vi "Circ Line Filter 2.vi"(5 "Filter On?":bool, 8 "error in":errorcluster, 11 "Data Cluster In":T1={"Display X"=[], "Display Y"=[], "Encoder"=[], "Phi Array"=[], "Active Channel"=0, "Raw X"=[], "Raw Y"=[], "IIR filter specifications"={"Topology"=enum."Butterworth", "Type"=enum."Lowpass", "Order"=1, "Lower Fc"=20.0, "Upper Fc"=200.0, "PB Ripple"=1.0, "SB Attenuation"=60.0}, "Sample Rate"=100.0, "optional IIR filter specifications"={"Lower PB"=100.0, "Upper PB"=0.0, "Lower SB"=200.0, "Upper SB"=0.0, "PB Gain"=-3.0, "SB Gain"=-60.0, "Scale"=TRUE}, "Display Select"=enum."Locations", "Cursor Position"=0.0, "Position Mark"=[], "Window Size"=0.0, "Last Active Channel"=0, "Rotate to:"=0.0, "Averaged Locations"=[], "Scale Factors"=[], "Filtered Data Measurements"={"Vpp"=0.0, "Phase"=0.0, "Slope"=0.0, "Start Point"={[], []}, "End Point"={[], []}, "Slope Points"={"x1"=0.0, "y1"=0.0, "x2"=0.0, "y2"=0.0}}, "Mp Flag"=FALSE, "Number of Channels"=0, "NormVals"=[], "Norm Buffer"=[], "Current Assignments"=[], "Current Filter Response"={"t0"=timestamp(0 s since 1904-01-01), "dt"=0.0, "Y"=[]}, "Filter Coeffs"=[], "Strip Data"=[], "X Display Null"=[], "Y Display Null"=[], "X Display Null Mod"=[], "Y Display Null Mod"=[], "file names"=[], "Current Data File"="", "Current Data Path"=path "", "Slide Value"=0, "Setup File Path"=path "", "Plot Color"=[], "Start Pts"=[], "End Pts"=[], "Slope Points"=[], "Raw Data Measurements"={"Vpp"=0.0, "Phase"=0.0, "Slope"=0.0, "Start Point"={[], []}, "End Point"={[], []}, "Slope Points"={"x1"=0.0, "y1"=0.0, "x2"=0.0, "y2"=0.0}}, "Raw Data"=refnum, "Calc X"=[], "Calc Y"=[], "3D X"=refnum, "3D Y"=refnum, "C/L Filter X  Waveforms"=[], "C/L Filter Y Waveforms"=[], "Command History"=[], "Filter Flag"={"Last Setter"="", "Status"=FALSE}, "Phi Array Scratch"=[], "Filetype"=enum."20\" Tool", "Channel List"={"Channel 1"=FALSE, "Channel 2"=FALSE, "Channel 3"=FALSE, "Channel 4"=FALSE, "Channel 5"=FALSE, "Channel 6"=FALSE, "Channel 7"=FALSE, "Channel 8"=FALSE, "Channel 9"=FALSE, "Channel 10"=FALSE, "Channel 11"=FALSE, "Channel 12"=FALSE, "Channel 13"=FALSE, "Channel 14"=FALSE, "Channel 15"=FALSE, "Channel 16"=FALSE, "Channel 17"=FALSE, "Channel 18"=FALSE, "Channel 19"=FALSE, "Channel 20"=FALSE, "Channel 21"=FALSE, "Channel 22"=FALSE, "Channel 23"=FALSE, "Channel 24"=FALSE, "Channel 25"=FALSE, "Channel 26"=FALSE, "Channel 27"=FALSE, "Channel 28"=FALSE, "Channel 29"=FALSE, "Channel 30"=FALSE, "Channel 31"=FALSE, "Channel 32"=FALSE}, "Channel Indicies"=[], "Calc Raw X"=[], "Calc Raw Y"=[], "Old Channel Indicies"=[]} {"Rotate to:" items=["1", "2", "3", "4", "5", "6", "7", "8", "9", "10", "11", "12", "3", "4", "15", "16", "17", "18", "19", "20", "21", "22", "23", "24"]; "Last Active Channel" items=["1", "2", "3", "4", "5", "6", "7", "8", "9", "10", "11", "12", "3", "4", "15", "16", "17", "18", "19", "20", "21", "22", "23", "24"]; "optional IIR filter specifications"."PB Gain" format="%0.2f"; "optional IIR filter specifications"."SB Gain" format="%0.2f"; "optional IIR filter specifications"."Lower SB" format="%0.2p"; "optional IIR filter specifications"."Upper SB" format="%0.2f"; "optional IIR filter specifications"."Lower PB" format="%0.2p"; "optional IIR filter specifications"."Upper PB" format="%0.2f"; "IIR filter specifications"."PB Ripple" format="%0.2f"; "IIR filter specifications"."Lower Fc" format="%0.2p"; "IIR filter specifications"."SB Attenuation" format="%0.2f"; "IIR filter specifications"."Upper Fc" format="%0.2p"; "Active Channel" items=["1", "2", "3", "4", "5", "6", "7", "8", "9", "10", "11", "12", "3", "4", "15", "16", "17", "18", "19", "20", "21", "22", "23", "24"]}) -> (0 "error out":errorcluster, 3 "Data Cluster Out":T1={"Display X"=[], "Display Y"=[], "Encoder"=[], "Phi Array"=[], "Active Channel"=0, "Raw X"=[], "Raw Y"=[], "IIR filter specifications"={"Topology"=enum."Butterworth", "Type"=enum."Lowpass", "Order"=1, "Lower Fc"=20.0, "Upper Fc"=200.0, "PB Ripple"=1.0, "SB Attenuation"=60.0}, "Sample Rate"=100.0, "optional IIR filter specifications"={"Lower PB"=100.0, "Upper PB"=0.0, "Lower SB"=200.0, "Upper SB"=0.0, "PB Gain"=-3.0, "SB Gain"=-60.0, "Scale"=TRUE}, "Display Select"=enum."Locations", "Cursor Position"=0.0, "Position Mark"=[], "Window Size"=0.0, "Last Active Channel"=0, "Rotate to:"=0.0, "Averaged Locations"=[], "Scale Factors"=[], "Filtered Data Measurements"={"Vpp"=0.0, "Phase"=0.0, "Slope"=0.0, "Start Point"={[], []}, "End Point"={[], []}, "Slope Points"={"x1"=0.0, "y1"=0.0, "x2"=0.0, "y2"=0.0}}, "Mp Flag"=FALSE, "Number of Channels"=0, "NormVals"=[], "Norm Buffer"=[], "Current Assignments"=[], "Current Filter Response"={"t0"=timestamp(0 s since 1904-01-01), "dt"=0.0, "Y"=[]}, "Filter Coeffs"=[], "Strip Data"=[], "X Display Null"=[], "Y Display Null"=[], "X Display Null Mod"=[], "Y Display Null Mod"=[], "file names"=[], "Current Data File"="", "Current Data Path"=path "", "Slide Value"=0, "Setup File Path"=path "", "Plot Color"=[], "Start Pts"=[], "End Pts"=[], "Slope Points"=[], "Raw Data Measurements"={"Vpp"=0.0, "Phase"=0.0, "Slope"=0.0, "Start Point"={[], []}, "End Point"={[], []}, "Slope Points"={"x1"=0.0, "y1"=0.0, "x2"=0.0, "y2"=0.0}}, "Raw Data"=refnum, "Calc X"=[], "Calc Y"=[], "3D X"=refnum, "3D Y"=refnum, "C/L Filter X  Waveforms"=[], "C/L Filter Y Waveforms"=[], "Command History"=[], "Filter Flag"={"Last Setter"="", "Status"=FALSE}, "Phi Array Scratch"=[], "Filetype"=enum."20\" Tool", "Channel List"={"Channel 1"=FALSE, "Channel 2"=FALSE, "Channel 3"=FALSE, "Channel 4"=FALSE, "Channel 5"=FALSE, "Channel 6"=FALSE, "Channel 7"=FALSE, "Channel 8"=FALSE, "Channel 9"=FALSE, "Channel 10"=FALSE, "Channel 11"=FALSE, "Channel 12"=FALSE, "Channel 13"=FALSE, "Channel 14"=FALSE, "Channel 15"=FALSE, "Channel 16"=FALSE, "Channel 17"=FALSE, "Channel 18"=FALSE, "Channel 19"=FALSE, "Channel 20"=FALSE, "Channel 21"=FALSE, "Channel 22"=FALSE, "Channel 23"=FALSE, "Channel 24"=FALSE, "Channel 25"=FALSE, "Channel 26"=FALSE, "Channel 27"=FALSE, "Channel 28"=FALSE, "Channel 29"=FALSE, "Channel 30"=FALSE, "Channel 31"=FALSE, "Channel 32"=FALSE}, "Channel Indicies"=[], "Calc Raw X"=[], "Calc Raw Y"=[], "Old Channel Indicies"=[]} {"Rotate to:" items=["1", "2", "3", "4", "5", "6", "7", "8", "9", "10", "11", "12", "3", "4", "15", "16", "17", "18", "19", "20", "21", "22", "23", "24"]; "Last Active Channel" items=["1", "2", "3", "4", "5", "6", "7", "8", "9", "10", "11", "12", "3", "4", "15", "16", "17", "18", "19", "20", "21", "22", "23", "24"]; "optional IIR filter specifications"."PB Gain" format="%0.2f"; "optional IIR filter specifications"."SB Gain" format="%0.2f"; "optional IIR filter specifications"."Lower SB" format="%0.2p"; "optional IIR filter specifications"."Upper SB" format="%0.2f"; "optional IIR filter specifications"."Lower PB" format="%0.2p"; "optional IIR filter specifications"."Upper PB" format="%0.2f"; "IIR filter specifications"."PB Ripple" format="%0.2f"; "IIR filter specifications"."Lower Fc" format="%0.2p"; "IIR filter specifications"."SB Attenuation" format="%0.2f"; "IIR filter specifications"."Upper Fc" format="%0.2p"; "Active Channel" items=["1", "2", "3", "4", "5", "6", "7", "8", "9", "10", "11", "12", "3", "4", "15", "16", "17", "18", "19", "20", "21", "22", "23", "24"]})   [LabVIEW 2017]
uses:
  <vilib>/Analysis/NI_AALPro.lvlib
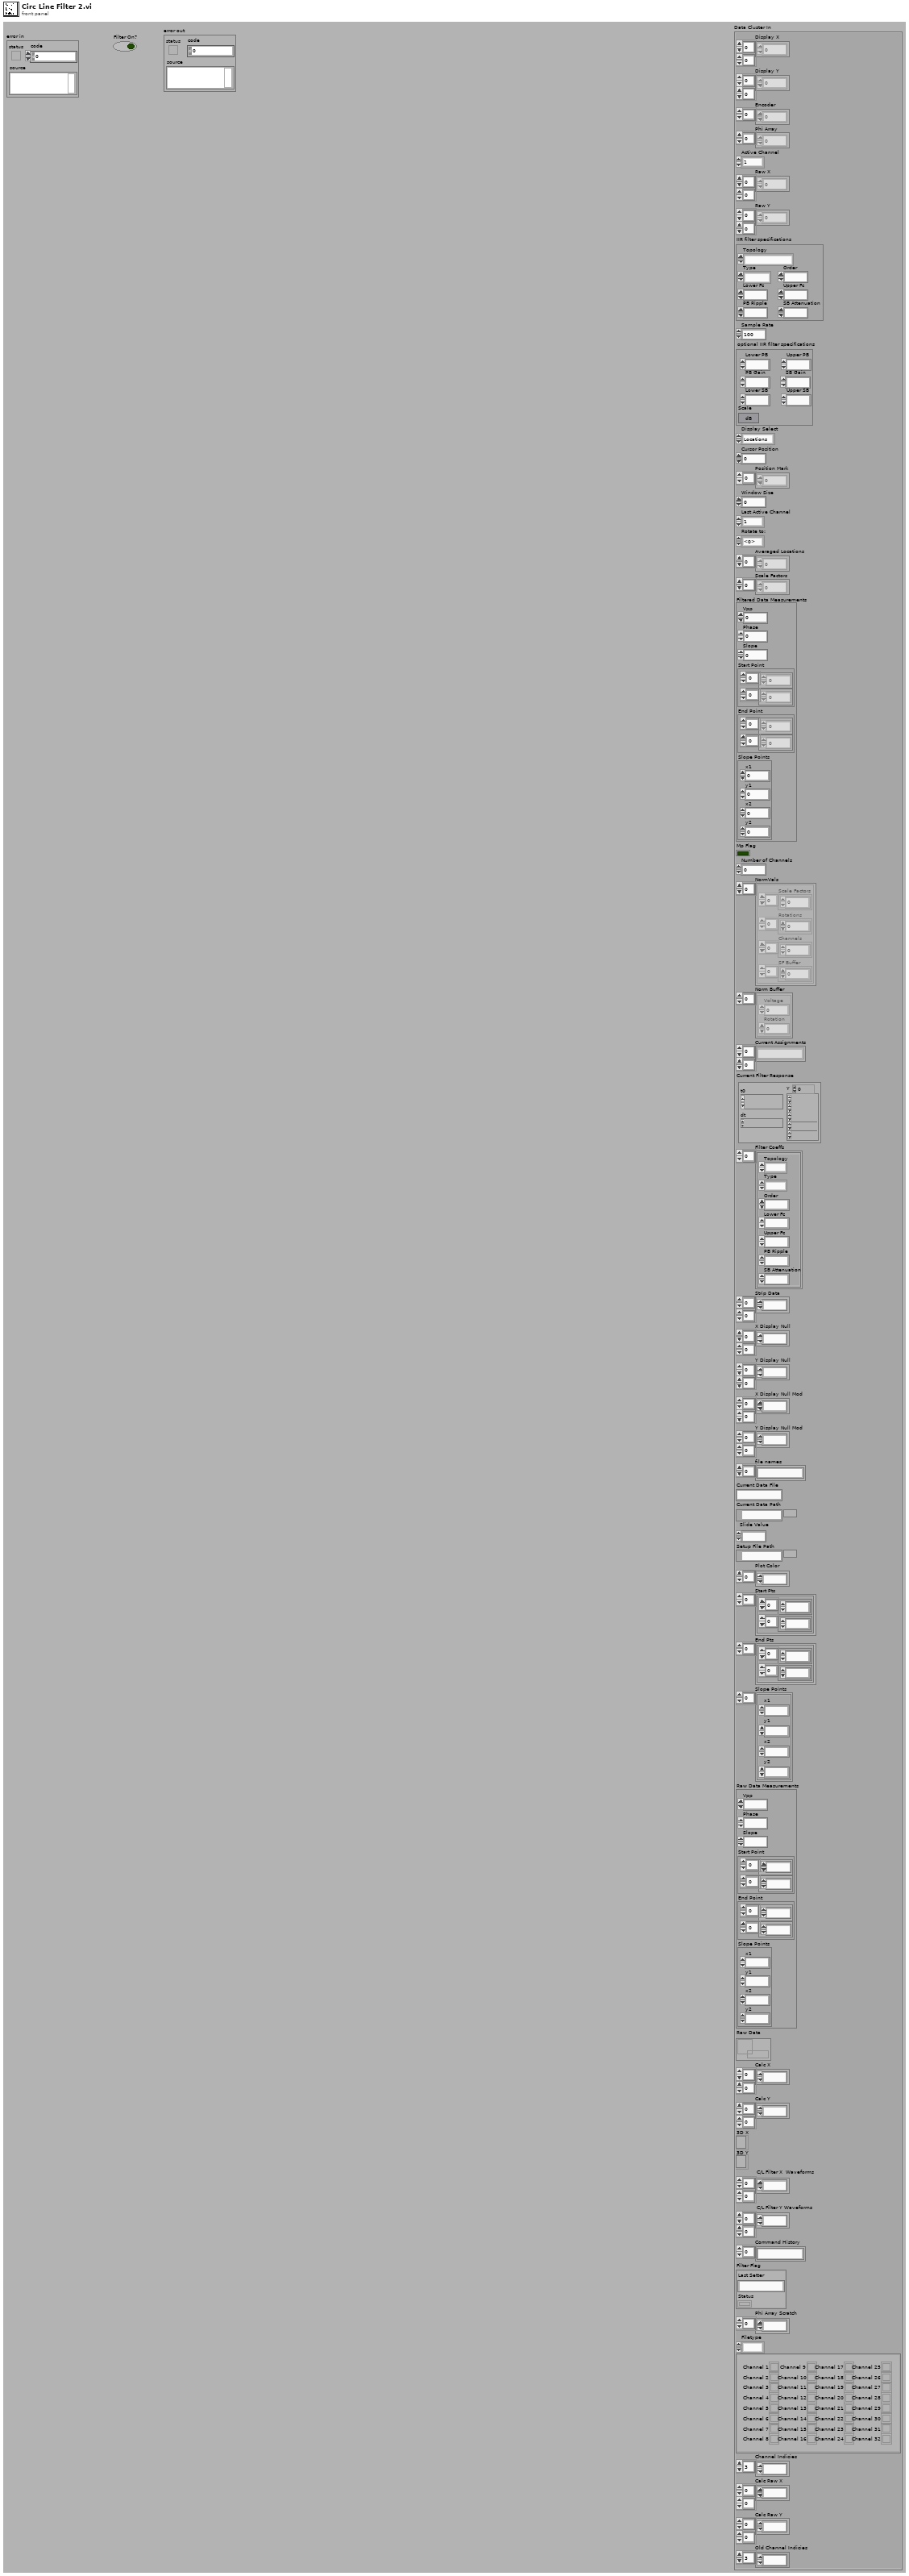
[diagram p1: front panel]
types:
  T1 = cluster{"Display X":dbl[][], "Display Y":dbl[][], "Encoder":dbl[], "Phi Array":dbl[], "Active Channel":i32, "Raw X":dbl[][], "Raw Y":dbl[][], "IIR filter specifications":cluster{"Topology":enum16{"Off", "Butterworth", "Chebyshev", "Inverse Chebyshev", "Elliptic", "Bessel"}, "Type":enum16{"Lowpass", "Highpass", "Bandpass", "Bandstop"}, "Order":i32, "Lower Fc":dbl, "Upper Fc":dbl, "PB Ripple":dbl, "SB Attenuation":dbl}, "Sample Rate":dbl, "optional IIR filter specifications":cluster{"Lower PB":dbl, "Upper PB":dbl, "Lower SB":dbl, "Upper SB":dbl, "PB Gain":dbl, "SB Gain":dbl, "Scale":bool}, "Display Select":enum32{"Channel Detail", "X Strip", "Y Strip", "Locations", "Contour", "3D", "Sorted"}, "Cursor Position":dbl, "Position Mark":sgl[], "Window Size":dbl, "Last Active Channel":i32, "Rotate to:":dbl, "Averaged Locations":i32[], "Scale Factors":dbl[], "Filtered Data Measurements":cluster{"Vpp":dbl, "Phase":dbl, "Slope":dbl, "Start Point":cluster{dbl[], dbl[]}, "End Point":cluster{dbl[], dbl[]}, "Slope Points":cluster{"x1":dbl, "y1":dbl, "x2":dbl, "y2":dbl}}, "Mp Flag":bool, "Number of Channels":i32, "NormVals":cluster{"Scale Factors":dbl[], "Rotations":dbl[], "Channels":i32[], "SF Buffer":dbl[]}[], "Norm Buffer":cluster{"Voltage":dbl, "Rotation":dbl}[], "Current Assignments":string[][], "Current Filter Response":waveform(dbl), "Filter Coeffs":cluster{"Topology":enum16{"Off", "Butterworth", "Chebyshev", "Inverse Chebyshev", "Elliptic", "Bessel"}, "Type":enum16{"Lowpass", "Highpass", "Bandpass", "Bandstop"}, "Order":i32, "Lower Fc":dbl, "Upper Fc":dbl, "PB Ripple":dbl, "SB Attenuation":dbl}[], "Strip Data":dbl[][], "X Display Null":dbl[][], "Y Display Null":dbl[][], "X Display Null Mod":dbl[][], "Y Display Null Mod":dbl[][], "file names":string[], "Current Data File":string, "Current Data Path":path, "Slide Value":i32, "Setup File Path":path, "Plot Color":i32[], "Start Pts":cluster{dbl[], dbl[]}[], "End Pts":cluster{dbl[], dbl[]}[], "Slope Points":cluster{"x1":dbl, "y1":dbl, "x2":dbl, "y2":dbl}[], "Raw Data Measurements":cluster{"Vpp":dbl, "Phase":dbl, "Slope":dbl, "Start Point":cluster{dbl[], dbl[]}, "End Point":cluster{dbl[], dbl[]}, "Slope Points":cluster{"x1":dbl, "y1":dbl, "x2":dbl, "y2":dbl}}, "Raw Data":refnum<queue>, "Calc X":dbl[][], "Calc Y":dbl[][], "3D X":refnum<k7>, "3D Y":refnum<k7>, "C/L Filter X  Waveforms":dbl[][], "C/L Filter Y Waveforms":dbl[][], "Command History":string[], "Filter Flag":cluster{"Last Setter":string, "Status":bool}, "Phi Array Scratch":dbl[], "Filetype":enum16{"20\" Tool", "24\"/36\" Tool"}, "Channel List":cluster{"Channel 1":bool, "Channel 2":bool, "Channel 3":bool, "Channel 4":bool, "Channel 5":bool, "Channel 6":bool, "Channel 7":bool, "Channel 8":bool, "Channel 9":bool, "Channel 10":bool, "Channel 11":bool, "Channel 12":bool, "Channel 13":bool, "Channel 14":bool, "Channel 15":bool, "Channel 16":bool, "Channel 17":bool, "Channel 18":bool, "Channel 19":bool, "Channel 20":bool, "Channel 21":bool, "Channel 22":bool, "Channel 23":bool, "Channel 24":bool, "Channel 25":bool, "Channel 26":bool, "Channel 27":bool, "Channel 28":bool, "Channel 29":bool, "Channel 30":bool, "Channel 31":bool, "Channel 32":bool}, "Channel Indicies":i32[], "Calc Raw X":dbl[][], "Calc Raw Y":dbl[][], "Old Channel Indicies":i32[]}
  T2 = enum32{"SVD", "Givens", "Givens2", "Householder", "LU Decomposition", "Cholesky"}
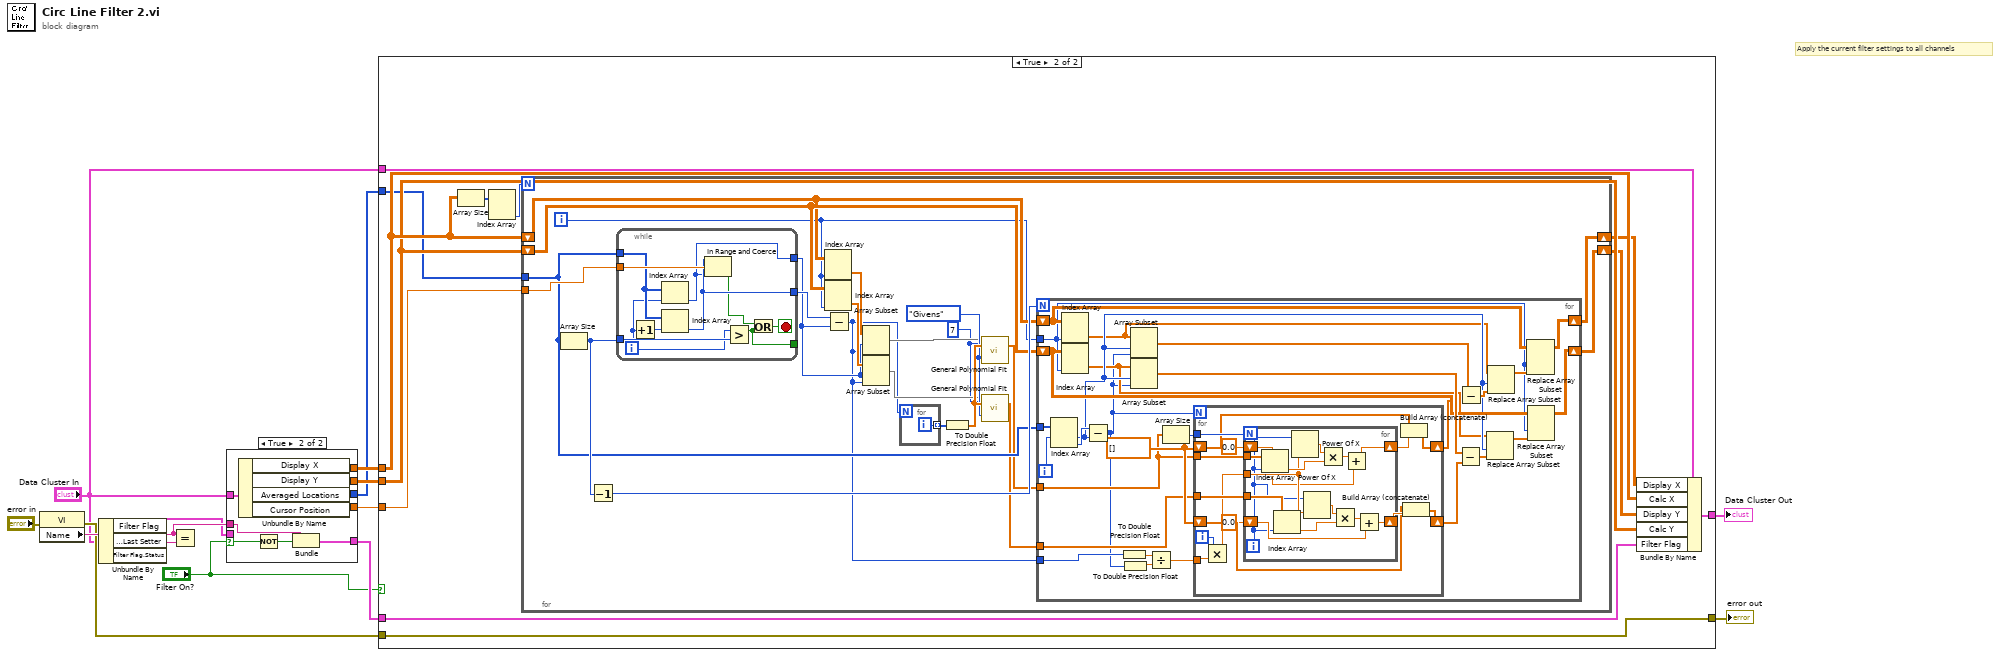
[diagram p0: block diagram]
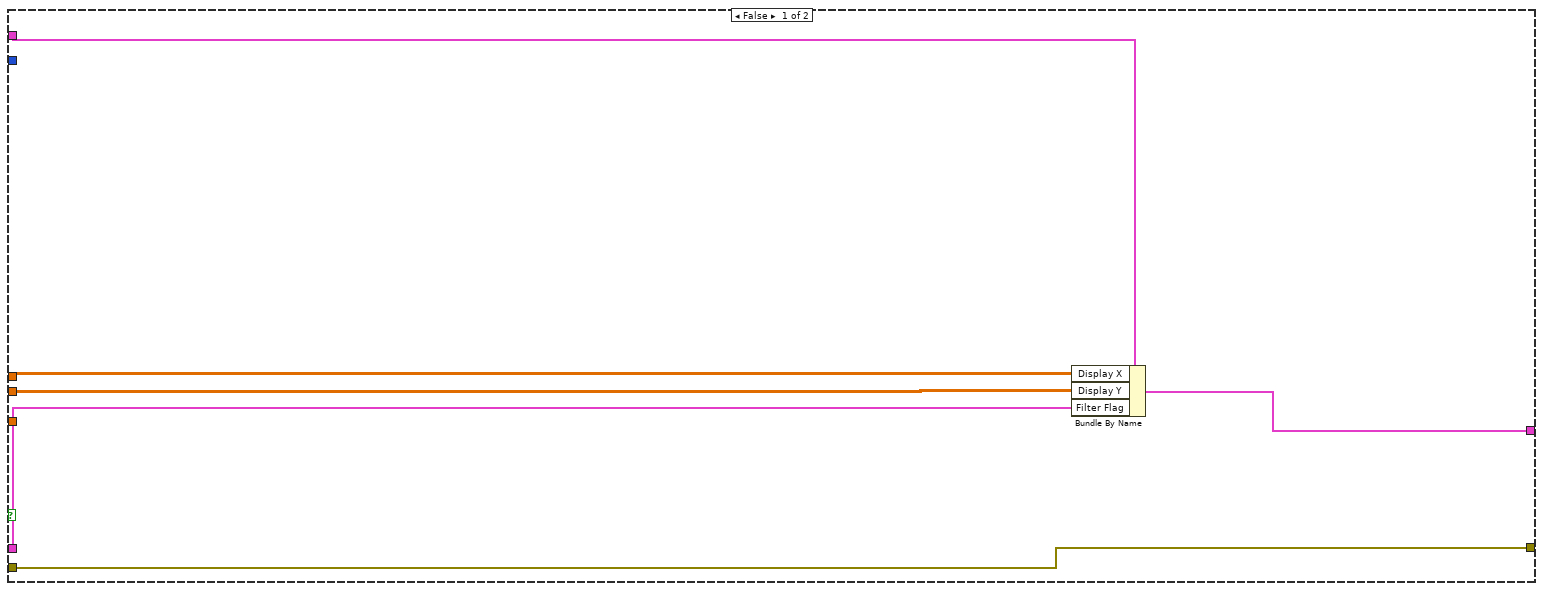
[diagram p2: hidden frame]
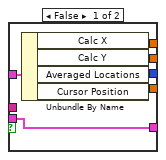
[diagram p3: hidden frame]
diagram:
  # "Apply the current filter settings to all channels"
  n1 = property class="VI"(error in="error in") -> (error out=w5:errorcluster, "Name"=w6:string)  [unwired: 1 in, 1 out]
  n2 = Unbundle By Name("Data Cluster In") -> ("Filter Flag"=w4:cluster{"Last Setter":string, "Status":bool}, "Filter Flag.Last Setter"=w8:string)  [unwired: 1 out]
  n3 = Equal?(x=w6, y=w8) -> ()  [unwired: 1 out]
  n4 = case shown="True" "Filter On?" {
    selector: "Filter On?" -> [_ w25]
    tunnel: "Data Cluster In" -> [w20 w29]
    tunnel: [w19 w28] -> w14
    tunnel: [w18 w27] -> w13
    tunnel: [w17 w26] -> w12
    tunnel: [w16 w21] -> w10
    tunnel: [w15 w22] -> w9
    tunnel: w6 -> [_ w24]
    tunnel: w4 -> [w15 _]
    frame False {
      n5 = Unbundle By Name(w20) -> ("Calc X"=w17:dbl[][], "Calc Y"=w18:dbl[][], "Averaged Locations"=w16:i32[], "Cursor Position"=w19:dbl)
    }
    frame True {
      n6 = Unbundle By Name(w29) -> ("Display X"=w26:dbl[][], "Display Y"=w27:dbl[][], "Averaged Locations"=w21:i32[], "Cursor Position"=w28:dbl)
      n7 = Not(x=w25) -> (.not. x?=w23:bool)
      n8 = Bundle("Name"=w24, w23) -> (w22:cluster{"Name":string, bool})  [unwired: 1 in]
    }
  }
  n9 = case shown="True" "Filter On?" {
    tunnel: w14 -> [_ w39]
    tunnel: w13 -> [w33 w41]
    tunnel: w12 -> [w34 w42]
    tunnel: [w35 w36] -> w11
    tunnel: w5 -> [w35 w36]
    tunnel: w10 -> [_ w40]
    tunnel: w9 -> [w31 w45]
    tunnel: "Data Cluster In" -> [w32 w47]
    tunnel: [w30 w46] -> w2
    frame False {
      n10 = Bundle By Name(cluster=w32, "Display X"=w34, "Display Y"=w33, "Filter Flag"=w31) -> (w30:T1)
    }
    frame True {
      n11 = Array Size(array=w42) -> (size(s)=w44:i32[])
      n12 = Index Array(array=w44) -> (element #2=w43:i32)  [unwired: 2 in, 1 out]
      n13 = for {
        N: w43 -> [_]
        tunnel: w39 -> [w69]
        tunnel: w40 -> [w57]
        shift-right: [w49] -> w38
        shift-left: w42 -> [w51]
        shift-right: [w48] -> w37
        shift-left: w41 -> [w56]
        i -> [w50]
        w66 = T2."Givens" ("algorithm")
        w60 = 7 ("polynomial order")
        n14 = Array Size(array=w57) -> (size(s)=w59:i32)
        n15 = Decrement(x=w59) -> (x-1=w58:i32)
        n16 = while {
          tunnel: w69 -> [w136]
          tunnel: w57 -> [w134]
          tunnel: [w132] -> w55
          tunnel: [w133] -> w61
          tunnel: w59 -> [w131]
          tunnel: [w127] -> _
          i -> [w130]
          stop <- w128 stop-if-true
          n17 = Increment(x=w130) -> (x+1=w135:i32)
          n18 = Index Array(array=w134, index=w130) -> (element=w132:i32)
          n19 = Index Array(array=w134, index=w135) -> (element=w133:i32)
          n20 = In Range and Coerce(upper limit=w133, x=w136, lower limit=w132) -> (In Range?=w129:bool)  [unwired: 1 out]
          n21 = Greater?(x=w130, y=w131) -> (0:w127:bool)
          n22 = Or(x=w129, y=w127) -> (x .or. y?=w128:bool)
        }
        n23 = Index Array(array=w51, index (col)=w50) -> (element=w62:dbl[])  [unwired: 1 in]
        n24 = Index Array(array=w56, index (col)=w50) -> (element=w63:dbl[])  [unwired: 1 in]
        n25 = Subtract(x=w61, y=w55) -> (x-y=w52:i32)
        n26 = Array Subset(array=w62, index=w55, length=w52) -> (w65:dbl[])
        n27 = Array Subset(array=w63, index=w55, length=w52) -> (w64:dbl[])
        n28 = for {
          N: w52 -> [_]
          tunnel: [w126] -> w68 mode=indexing
          i -> [w126]
        }
        n29 = To Double Precision Float(number=w68) -> (double precision float=w67:dbl[])
        n30 = call <vilib>:"General Polynomial Fit.vi"("Y"=w65, "polynomial order"=w60, "X"=w67, "algorithm"=w66) -> ("Polynomial Coefficients"=w54:dbl[])  [unwired: 8 in, 3 out]
        n31 = call <vilib>:"General Polynomial Fit.vi"("Y"=w64, "polynomial order"=w60, "X"=w67, "algorithm"=w66) -> ("Polynomial Coefficients"=w53:dbl[])  [unwired: 8 in, 3 out]
        n32 = for {
          N: w58 -> [_]
          tunnel: w57 -> [w97]
          tunnel: w50 -> [w83]
          shift-right: [w86] -> w49
          shift-left: w51 -> [w88]
          shift-right: [w85] -> w48
          shift-left: w56 -> [w87]
          tunnel: w54 -> [w78]
          tunnel: w53 -> [w77]
          tunnel: w52 -> [w71]
          i -> [w96]
          w80 = dbl[] []
          n33 = Index Array(array=w97, index #1=w96) -> (element #1=w84:i32, element #2=w95:i32)  [unwired: 1 in]
          n34 = Index Array(array=w88, index (col)=w83) -> (element=w81:dbl[])  [unwired: 1 in]
          n35 = Index Array(array=w87, index (col)=w83) -> (element=w82:dbl[])  [unwired: 1 in]
          n36 = Subtract(x=w95, y=w84) -> (x-y=w70:i32)
          n37 = To Double Precision Float(number=w71) -> (double precision float=w73:dbl)
          n38 = To Double Precision Float(number=w70) -> (double precision float=w72:dbl)
          n39 = Array Subset(array=w81, index=w84, length=w70) -> (w92:dbl[])
          n40 = Array Subset(array=w82, index=w84, length=w70) -> (w89:dbl[])
          n41 = Divide(x=w73, y=w72) -> (x/y=w76:dbl)
          n42 = Array Size(array=w78) -> (size(s)=w79:i32)
          n43 = for {
            N: w70 -> [_]
            tunnel: w77 -> [w109]
            tunnel: w78 -> [w111]
            tunnel: w79 -> [w110]
            shift-right: [w108] -> w74
            shift-left: w80 -> [w107]
            shift-right: [w104] -> w75
            shift-left: w80 -> [w103]
            tunnel: w76 -> [w100]
            i -> [w99]
            n44 = Multiply(x=w99, y=w100) -> (x*y=w98:dbl)
            n45 = for {
              N: w110 -> [_]
              tunnel: w98 -> [w114]
              tunnel: w111 -> [w123]
              shift-right: [w124] -> w106
              shift-left: 0.0 -> [w112]
              tunnel: w109 -> [w115]
              shift-right: [w117] -> w105
              shift-left: 0.0 -> [w116]
              i -> [w113]
              n46 = Index Array(array=w123, index=w113) -> (element=w121:dbl)
              n47 = Index Array(array=w115, index=w113) -> (element=w120:dbl)
              n48 = Power Of X(1:w114, 2:w113) -> (0:w122:dbl)
              n49 = Power Of X(1:w114, 2:w113) -> (0:w119:dbl)
              n50 = Multiply(x=w122, y=w121) -> (x*y=w125:dbl)
              n51 = Multiply(x=w119, y=w120) -> (x*y=w118:dbl)
              n52 = Add(x=w125, y=w112) -> (x+y=w124:dbl)
              n53 = Add(x=w118, y=w116) -> (x+y=w117:dbl)
            }
            n54 = Build Array (concatenate)(w107, w106) -> (w108:dbl[])
            n55 = Build Array (concatenate)(w103, w105) -> (w104:dbl[])
          }
          n56 = Subtract(x=w89, y=w75) -> (x-y=w91:dbl[])
          n57 = Subtract(x=w92, y=w74) -> (x-y=w93:dbl[])
          n58 = Replace Array Subset(array=w82, new element=w91, index=w84) -> (w90:dbl[])
          n59 = Replace Array Subset(array=w81, new element=w93, index=w84) -> (w94:dbl[])
          n60 = Replace Array Subset(array=w88, new element=w94, index (col)=w83) -> (w86:dbl[][])  [unwired: 1 in]
          n61 = Replace Array Subset(array=w87, new element=w90, index (col)=w83) -> (w85:dbl[][])  [unwired: 1 in]
        }
      }
      n62 = Bundle By Name(cluster=w47, "Display X"=w38, "Calc X"=w42, "Display Y"=w37, "Calc Y"=w41, "Filter Flag"=w45) -> (w46:T1)
    }
  }
  "error out" <- w11
  "Data Cluster Out" <- w2
